vi "Compare Values.vi"(6 "Compare Window":dbl, 10 "Value2 In":dbl, 11 "Value1 In":dbl) -> (2 "Delta Out":dbl, 3 "Within Window?":bool)   [LabVIEW 2015]
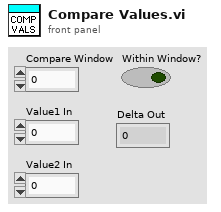
[diagram p1: front panel]
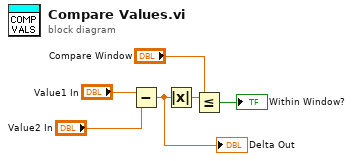
[diagram p0: block diagram]
diagram:
  n1 = Subtract(x="Value1 In", y="Value2 In") -> (x-y=w5:dbl)
  "Delta Out" <- w5
  n2 = Absolute Value(x=w5) -> (abs(x)=w1:dbl)
  n3 = Less Or Equal?(x=w1, y="Compare Window") -> (x <= y?=→"Within Window?":bool)
